vi "ULx Read (Counter DBL 1Chan 1Samp).vi"(0 "task in":refnum<k24>, 9 "timeout":dbl=10.0, 11 "error in":errorcluster) -> (4 "task out":refnum<k24>, 6 "data":dbl format="%_6g", 15 "error out":errorcluster)   [LabVIEW 2020]
doc: "Reads a single floating-point sample from a task that contains a single counter input."
uses:
  C:/Users/William/Documents/LV 2020 builds/LeaktestDAQ/Source-v33/ULx_LV.dll
  ULx_LV.dll
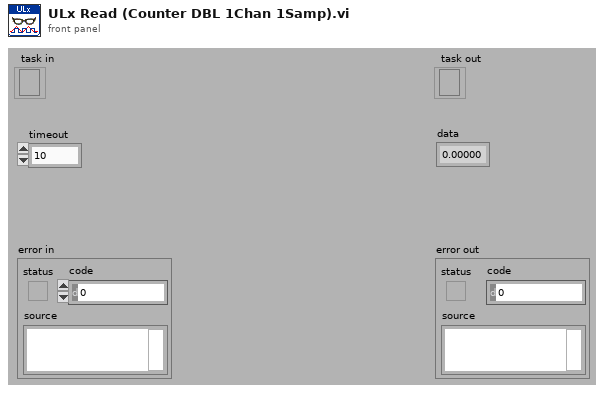
[diagram p1: front panel]
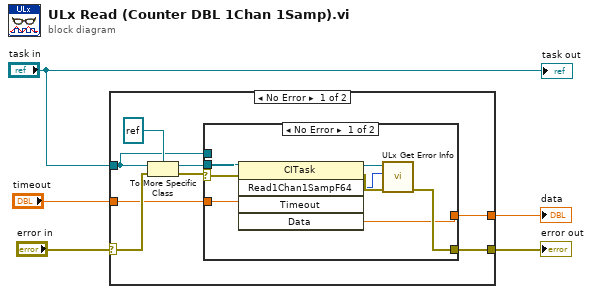
[diagram p0: block diagram]
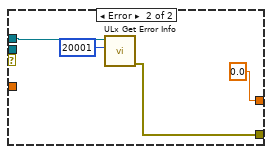
[diagram p2: hidden frame]
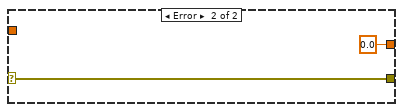
[diagram p3: hidden frame]
diagram:
  n1 = case shown="No Error" "error in" {
    selector: "error in" -> [w13 w26]
    tunnel: "task in" -> [w6 _]
    tunnel: "timeout" -> [w9 _]
    tunnel: [w8 0.0 ("Read1Chan1SampF64")] -> w3
    tunnel: [w7 w26] -> w2
    frame No Error {
      n2 = To More Specific Class(target class=refnum<k24> refnum, reference=w6, error in=w13) -> (specific class reference=w10:refnum<k24>, error out=w11:errorcluster)
      n3 = case shown="No Error" w11 {
        selector: w11 -> [w20 _]
        tunnel: w10 -> [w21 _]
        tunnel: w9 -> [w19 _]
        tunnel: [w15 0.0 ("Read1Chan1SampF64")] -> w8
        tunnel: [w16 w22] -> w7
        tunnel: w6 -> [_ w24]
        frame No Error {
          n4 = invoke class="CITask" method="Read1Chan1SampF64"(reference=w21, error in=w20, "Timeout"=w19) -> (reference out=w17:refnum<k24>, error out=w18:errorcluster, "Read1Chan1SampF64"=w14:i32, "Data"=w15:dbl)  [unwired: 2 in, 1 out]
          n5 = call "ULx Get Error Info.vi"("error in"=w18, "ErrorCode"=w14, "task in"=w17) -> ("error out"=w16:errorcluster)  [unwired: 8 in]
        }
        frame Error {
          n6 = call "ULx Get Error Info.vi"("ErrorCode"=20001, "task in"=w24) -> ("error out"=w22:errorcluster)  [unwired: 9 in]
        }
      }
    }
    frame Error {
    }
  }
  "data" <- w3
  "error out" <- w2
  "task out" <- "task in"
